vi "UpdateMovingAverages.vi"(7 "FilteredAndRectified":waveform(dbl)[](graph) caption="Filtered\nand\nRectified", 8 "mvcSize":dbl=300.0 caption="Upper Cut-Off", 9 "dispSize":dbl=20.0 caption="Lower Cut-Off", 10 "MVC Data":cluster{"queue out":refnum<queue>, dbl, dbl}[](array[cluster]), 11 "Disp Data":cluster{"queue out":refnum<queue>, dbl, dbl}[](array[cluster])) -> (2 "MVC Data Out":cluster{"queue out":refnum<queue>, dbl, dbl}[](array[cluster]), 3 "Disp Data Out":cluster{"queue out":refnum<queue>, dbl, dbl}[](array[cluster]))   [LabVIEW 2016]
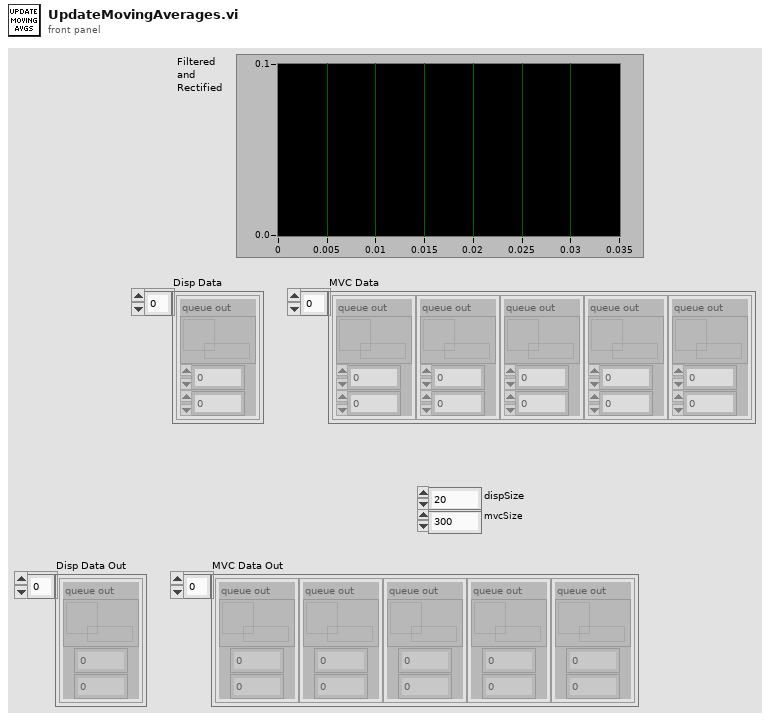
[diagram p1: front panel]
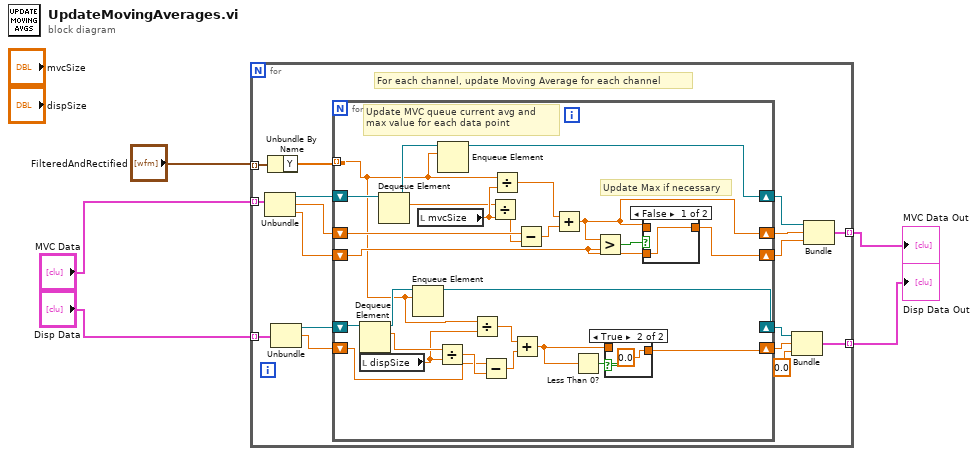
[diagram p0: block diagram]
diagram:
  n1 = for {
    tunnel: "FilteredAndRectified" -> [w22] mode=indexing
    tunnel: "MVC Data" -> [w20] mode=indexing
    tunnel: [w14] -> w2 mode=indexing
    tunnel: "Disp Data" -> [w12] mode=indexing
    tunnel: [w7] -> w1 mode=indexing
    # "For each channel, update Moving Average for each channel"
    n2 = Unbundle(w20) -> ("queue out"=w13:refnum<queue>, w19:dbl, w18:dbl)
    n3 = Unbundle By Name(w22) -> ("Y"=w21:dbl[])
    n4 = Unbundle(w12) -> ("queue out"=w9:refnum<queue>, w6:dbl)  [unwired: 1 out]
    n5 = for {
      tunnel: w21 -> [w31] mode=indexing
      shift-right: [w36] -> w16
      shift-left: w19 -> [w48]
      shift-right: [w40] -> w17
      shift-left: w13 -> [w39]
      shift-right: [w42] -> w15
      shift-left: w18 -> [w41]
      shift-right: [w25] -> w10
      shift-left: w6 -> [w23]
      shift-right: [w33] -> w11
      shift-left: w9 -> [w27]
      # "Update Max if necessary"
      # "Update MVC queue current avg and \nmax value for each data point"
      n6 = Dequeue Element(queue=w27) -> (queue out=w35:refnum<queue>, element=w34:dbl)  [unwired: 2 in, 2 out]
      n7 = local read "dispSize"() -> (w32:dbl)
      n8 = Dequeue Element(queue=w39) -> (queue out=w38:refnum<queue>, element=w37:dbl)  [unwired: 2 in, 2 out]
      n9 = Enqueue Element(queue=w35, element=w31) -> (queue out=w33:refnum<queue>)  [unwired: 2 in, 2 out]
      n10 = local read "mvcSize"() -> (w46:dbl)
      n11 = Divide(x=w34, y=w32) -> (x/y=w30:dbl)
      n12 = Enqueue Element(queue=w38, element=w31) -> (queue out=w40:refnum<queue>)  [unwired: 2 in, 2 out]
      n13 = Divide(x=w31, y=w32) -> (x/y=w29:dbl)
      n14 = Subtract(x=w23, y=w30) -> (x-y=w28:dbl)
      n15 = Divide(x=w37, y=w46) -> (x/y=w47:dbl)
      n16 = Divide(x=w31, y=w46) -> (x/y=w44:dbl)
      n17 = Add(x=w29, y=w28) -> (x+y=w24:dbl)
      n18 = Subtract(x=w48, y=w47) -> (x-y=w45:dbl)
      n19 = Add(x=w44, y=w45) -> (x+y=w36:dbl)
      n20 = Less Than 0?(x=w24) -> (x < 0?=w26:bool)
      n21 = Greater?(x=w36, y=w41) -> (0:w43:bool)
      n22 = case shown="True" w26 {
        tunnel: [w49 0.0] -> w25
        tunnel: w24 -> [w49 _]
        frame False {
        }
        frame True {
        }
      }
      n23 = case shown="False" w43 {
        tunnel: w36 -> [_ w52]
        tunnel: [w51 w52] -> w42
        tunnel: w41 -> [w51 _]
        frame False {
        }
        frame True {
        }
      }
    }
    n24 = Bundle("queue out"=w11, w10, 0.0) -> (w7:cluster{"queue out":refnum<queue>, dbl, dbl})  [unwired: 1 in]
    n25 = Bundle("queue out"=w17, w16, w15) -> (w14:cluster{"queue out":refnum<queue>, dbl, dbl})  [unwired: 1 in]
  }
  "MVC Data Out" <- w2
  "Disp Data Out" <- w1
